vi "AD5781Init.vi"() -> (1 "WriteEqualsRead":bool, 3 "Readback":u32)   [LabVIEW 2014]
uses:
  Controls/FPGA SPI_FPGA SPI State.ctl
  <vilib>/rvi/eio/common/nirviEmuTemplateMethod_errors.vi
  <vilib>/rvi/Emulation/niFpgaSctlEmulationGetInTimedLoop.vi
  Code/FPGA SPI_Globals.vi
  <vilib>/rvi/Emulation/niFpgaProcessEmulError.vi
  <vilib>/rvi/Emulation/niFpgaGetClockAttributes.vi
  <vilib>/rvi/Emulation/niFpgaEmulationReportErrorSimple.vi
  <vilib>/rvi/Emulation/niFpgaCriticalErrorInLSC.vi
  <vilib>/eio/EIONode/EIONode.xnode
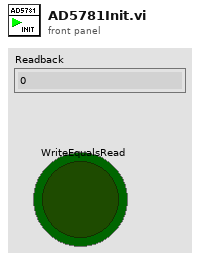
[diagram p1: front panel]
types:
  T1 = typedef "FPGA SPI_FPGA SPI State.ctl" = enum8{"Idle", "Read/Write SPI", "Configure"}
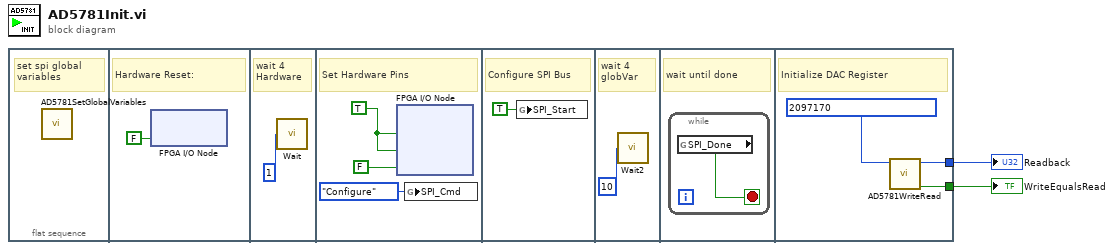
[diagram p0: block diagram]
diagram:
  n1 = flat-sequence {
    tunnel: [w12] -> w2
    tunnel: [w11] -> w1
    frame #0 {
      # "set spi global variables"
      n2 = call "AD5781SetGlobalVariables.vi"() -> ()  [unwired: 12 in]
    }
    frame #1 {
      # "Hardware Reset:"
      n3 = xnode "FPGA I/O Node"("RESET"=FALSE) -> ()  [unwired: 1 in, 1 out]
    }
    frame #2 {
      # "wait 4\nHardware"
      n4 = call "Wait"("Count(uSec)"=u8 1) -> ()  [unwired: 1 out]
    }
    frame #3 {
      w7 = TRUE ("CLR")
      # "Set Hardware Pins"
      n5 = xnode "FPGA I/O Node"("CLR"=w7, "RESET"=w7, "LDAC"=FALSE ("CLR")) -> ()  [unwired: 3 in, 3 out]
      n6 = global write "FPGA SPI_Globals.vi" "SPI_Cmd"(FPGA_SPI_FPGA_SPI_State."Configure" ("SPI_Cmd")) -> ()
    }
    frame #4 {
      # "Configure SPI Bus"
      n7 = global write "FPGA SPI_Globals.vi" "SPI_Start"(TRUE ("SPI_Start")) -> ()
    }
    frame #5 {
      # "wait 4\nglobVar"
      n8 = call "Wait2"("Count(Ticks)"=u8 10 ("Count(uSec)")) -> ()  [unwired: 1 out]
    }
    frame #6 {
      # "wait until done"
      n9 = while {
        stop <- w10 stop-if-true
        n10 = global read "FPGA SPI_Globals.vi" "SPI_Done"() -> (w10:bool)
      }
    }
    frame #7 {
      # "Initialize DAC Register"
      n11 = call "AD5781WriteRead.vi"("Write"=u32 2097170 ("U32")) -> ("WriteEqualsRead"=w11:bool, "Readback"=w12:u32)  [unwired: 6 in]
    }
  }
  "Readback" <- w2
  "WriteEqualsRead" <- w1
